vi "DisableScreenSaver.vi"(8 "No Error":errorcluster) -> (0 "Error Out":errorcluster)   [LabVIEW 2026, in "SDL3.lvlib" / "Video.lvlib"]
doc: "<B>Summary</B>\nPrevent the screen from being blanked by a screen saver.\n\n<B>Remarks</B>\nIf you disable the screensaver, it is automatically re-enabled when SDL quits.\n\nThe screensaver is disabled by default, but this may by changed by <B>SDL_HINT_VIDEO_ALLOW_SCREENSAVER</B>."
uses:
  Video.lvlib
  <vilib>/Utility/error.llb/Error Cluster From Error Code.vi
  Error/Error.lvlib
  Lib/SDL3.dll
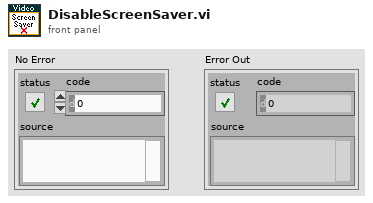
[diagram p1: front panel]
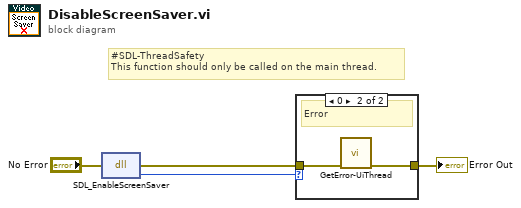
[diagram p0: block diagram]
diagram:
  # "#SDL-ThreadSafety\nThis function should only be called on the main thread."
  n1 = dll-call lib="C:/Users/saukko/Dev/LV-SDL3/Sources/SDL3/Lib/SDL3.*" fn="SDL_EnableScreenSaver"(error in="No Error") -> (error out=w2:errorcluster, "return type"=w1:i32)  [unwired: 2 in, 1 out]
  n2 = case shown="0" w1 {
    tunnel: w2 -> [w5 w7]
    tunnel: [w5 w6] -> w3
    frame Default {
      # "Ok"
    }
    frame 0 {
      # "Error"
      n3 = call "GetError-UiThread.vi"("No Error"=w7) -> ("error out"=w6:errorcluster)  [unwired: 10 in]
    }
  }
  "Error Out" <- w3
